vi "Configure SMU.vi"(5 "aperture time":dbl=0.001, 7 "Source Mode":enum16{"Voltage", "Current"}(ring), 8 "error in (no error)":errorcluster, 9 "Settings":T2 {"Sense" items=["Local"=1008, "Remote"=1009]}, 10 "Pins":string[](array[string]), 11 "Semiconductor Module Context":T3) -> (0 "error out":errorcluster)   [LabVIEW 2013]
uses:
  <vilib>/NI_TestStand_SemiconductorModule/NI_TestStand_Semiconductor_Module.lvlibp/PinMap/General/SemiconductorModuleContext.ctl
  <instrlib>/niDCPower/nidcpower.llb/niDCPower Sense.ctl
  <instrlib>/niDCPower/nidcpower.llb/niDCPower Aperture Time Units.ctl
  <instrlib>/niDCPower/nidcpower.llb/niDCPower Output Function.ctl
  <vilib>/NI_TestStand_SemiconductorModule/NI_TestStand_Semiconductor_Module.lvlibp/PinMap/DC Power/PinsToNIDCPowerSessions.vi
  <vilib>/NI_TestStand_SemiconductorModule/NI_TestStand_Semiconductor_Module.lvlibp
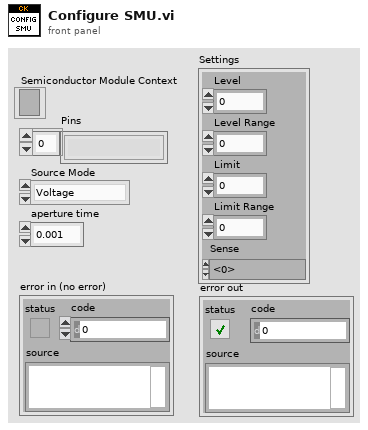
[diagram p1: front panel]
types:
  T1 = typedef "niDCPower Sense.ctl" = i32
  T2 = cluster{"Level":dbl, "Level Range":dbl, "Limit":dbl, "Limit Range":dbl, "Sense":T1}
  T3 = typedef "NI_TestStand_Semiconductor_Module.lvlibp/SemiconductorModuleContext.ctl" = refnum<k7>
  T4 = typedef "niDCPower Aperture Time Units.ctl" = i32
  T5 = typedef "niDCPower Output Function.ctl" = i32
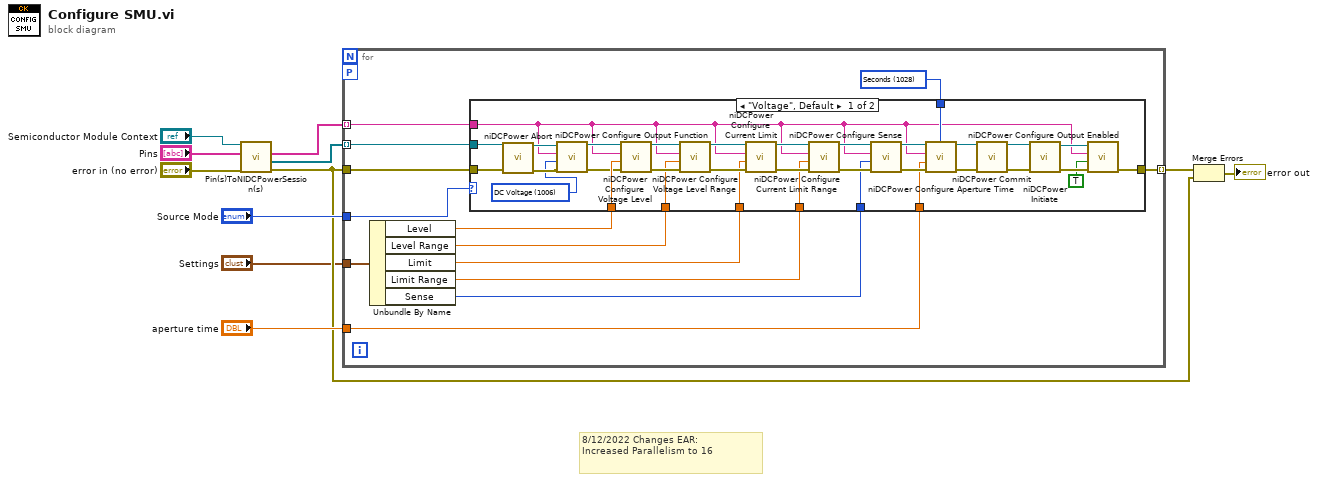
[diagram p0: block diagram]
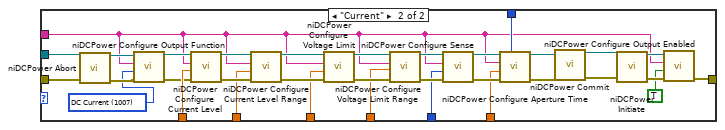
[diagram p2: hidden frame]
diagram:
  # "8/12/2022 Changes EAR:\nIncreased Parallelism to 16"
  n1 = call-poly <vilib>:"Pin(s)ToNIDCPowerSession(s).vi"("error in (no error)"="error in (no error)", "Pins"="Pins", "Semiconductor Module Context"="Semiconductor Module Context") -> ("error out"=w3:errorcluster, "Instrument Sessions"=w9:refnum<k15>[], "Channel Lists"=w8:string[])  [unwired: 4 in, 2 out]
  n2 = for {
    tunnel: w9 -> [w23] mode=indexing
    tunnel: w8 -> [w22] mode=indexing
    tunnel: "Settings" -> [w20]
    tunnel: "Source Mode" -> [w15]
    tunnel: "aperture time" -> [w12]
    tunnel: w3 -> [w24]
    tunnel: [w21] -> w5 mode=indexing
    workers-P: _ -> [_]
    w13 = T4 1028 items=["Seconds"=1028, "Powerline Cycles"=1029] ("aperture time units")
    n3 = Unbundle By Name(w20) -> ("Level"=w19:dbl, "Level Range"=w18:dbl, "Limit"=w17:dbl, "Limit Range"=w16:dbl, "Sense"=w14:T1)
    n4 = case shown="\"Voltage\", Default" w15 {
      tunnel: w24 -> [w31 w73]
      tunnel: w23 -> [w33 w72]
      tunnel: w22 -> [w26 w59]
      tunnel: [w28 w60] -> w21
      tunnel: w19 -> [w49 w90]
      tunnel: w18 -> [w48 w87]
      tunnel: w17 -> [w47 w84]
      tunnel: w16 -> [w46 w81]
      tunnel: w14 -> [w41 w78]
      tunnel: w12 -> [w43 w75]
      tunnel: w13 -> [w42 w74]
      frame "Voltage", Default {
        w34 = T5 1006 items=["DC Voltage"=1006, "DC Current"=1007, "Pulse Voltage"=1049, "Pulse Current"=1050] ("output function")
        n5 = call <instrlib>:"niDCPower Abort.vi"("error in (no error)"=w31, "instrument handle"=w33) -> ("error out"=w36:errorcluster, "instrument handle out"=w35:refnum<k15>)  [unwired: 8 in]
        n6 = call <instrlib>:"niDCPower Configure Output Function.vi"("error in (no error)"=w36, "output function"=w34, "channel name"=w26, "instrument handle"=w35) -> ("error out"=w30:errorcluster, "instrument handle out"=w32:refnum<k15>)  [unwired: 6 in]
        n7 = call <instrlib>:"niDCPower Configure Voltage Level.vi"("error in (no error)"=w30, "voltage level"=w49, "channel name"=w26, "instrument handle"=w32) -> ("error out"=w57:errorcluster, "instrument handle out"=w56:refnum<k15>)  [unwired: 6 in]
        n8 = call <instrlib>:"niDCPower Configure Voltage Level Range.vi"("error in (no error)"=w57, "voltage level range"=w48, "channel name"=w26, "instrument handle"=w56) -> ("error out"=w55:errorcluster, "instrument handle out"=w53:refnum<k15>)  [unwired: 6 in]
        n9 = call <instrlib>:"niDCPower Configure Current Limit.vi"("error in (no error)"=w55, "current limit"=w47, "channel name"=w26, "instrument handle"=w53) -> ("error out"=w54:errorcluster, "instrument handle out"=w52:refnum<k15>)  [unwired: 6 in]
        n10 = call <instrlib>:"niDCPower Configure Current Limit Range.vi"("error in (no error)"=w54, "current limit range"=w46, "channel name"=w26, "instrument handle"=w52) -> ("error out"=w51:errorcluster, "instrument handle out"=w50:refnum<k15>)  [unwired: 6 in]
        n11 = call <instrlib>:"niDCPower Configure Sense.vi"("error in (no error)"=w51, "sense"=w41, "channel name"=w26, "instrument handle"=w50) -> ("error out"=w45:errorcluster, "instrument handle out"=w44:refnum<k15>)  [unwired: 6 in]
        n12 = call <instrlib>:"niDCPower Configure Aperture Time.vi"("aperture time units"=w42, "error in (no error)"=w45, "aperture time"=w43, "channel name"=w26, "instrument handle"=w44) -> ("error out"=w39:errorcluster, "instrument handle out"=w40:refnum<k15>)  [unwired: 5 in]
        n13 = call <instrlib>:"niDCPower Commit.vi"("error in (no error)"=w39, "instrument handle"=w40) -> ("error out"=w38:errorcluster, "instrument handle out"=w37:refnum<k15>)  [unwired: 8 in]
        n14 = call <instrlib>:"niDCPower Initiate.vi"("error in (no error)"=w38, "instrument handle"=w37) -> ("error out"=w29:errorcluster, "instrument handle out"=w27:refnum<k15>)  [unwired: 8 in]
        n15 = call <instrlib>:"niDCPower Configure Output Enabled.vi"("error in (no error)"=w29, "output enabled"=TRUE, "channel name"=w26, "instrument handle"=w27) -> ("error out"=w28:errorcluster)  [unwired: 6 in, 1 out]
      }
      frame "Current" {
        w67 = T5 1007 items=["DC Voltage"=1006, "DC Current"=1007, "Pulse Voltage"=1049, "Pulse Current"=1050] ("output function")
        n16 = call <instrlib>:"niDCPower Abort.vi"("error in (no error)"=w73, "instrument handle"=w72) -> ("error out"=w69:errorcluster, "instrument handle out"=w68:refnum<k15>)  [unwired: 8 in]
        n17 = call <instrlib>:"niDCPower Configure Output Function.vi"("error in (no error)"=w69, "output function"=w67, "channel name"=w59, "instrument handle"=w68) -> ("error out"=w71:errorcluster, "instrument handle out"=w70:refnum<k15>)  [unwired: 6 in]
        n18 = call <instrlib>:"niDCPower Configure Current Level.vi"("error in (no error)"=w71, "current level"=w90, "channel name"=w59, "instrument handle"=w70) -> ("error out"=w89:errorcluster, "instrument handle out"=w88:refnum<k15>)  [unwired: 6 in]
        n19 = call <instrlib>:"niDCPower Configure Current Level Range.vi"("error in (no error)"=w89, "current level range"=w87, "channel name"=w59, "instrument handle"=w88) -> ("error out"=w86:errorcluster, "instrument handle out"=w85:refnum<k15>)  [unwired: 6 in]
        n20 = call <instrlib>:"niDCPower Configure Voltage Limit.vi"("error in (no error)"=w86, "voltage limit"=w84, "channel name"=w59, "instrument handle"=w85) -> ("error out"=w83:errorcluster, "instrument handle out"=w82:refnum<k15>)  [unwired: 6 in]
        n21 = call <instrlib>:"niDCPower Configure Voltage Limit Range.vi"("error in (no error)"=w83, "voltage limit range"=w81, "channel name"=w59, "instrument handle"=w82) -> ("error out"=w80:errorcluster, "instrument handle out"=w79:refnum<k15>)  [unwired: 6 in]
        n22 = call <instrlib>:"niDCPower Configure Sense.vi"("error in (no error)"=w80, "sense"=w78, "channel name"=w59, "instrument handle"=w79) -> ("error out"=w77:errorcluster, "instrument handle out"=w76:refnum<k15>)  [unwired: 6 in]
        n23 = call <instrlib>:"niDCPower Configure Aperture Time.vi"("aperture time units"=w74, "error in (no error)"=w77, "aperture time"=w75, "channel name"=w59, "instrument handle"=w76) -> ("error out"=w66:errorcluster, "instrument handle out"=w65:refnum<k15>)  [unwired: 5 in]
        n24 = call <instrlib>:"niDCPower Commit.vi"("error in (no error)"=w66, "instrument handle"=w65) -> ("error out"=w63:errorcluster, "instrument handle out"=w64:refnum<k15>)  [unwired: 8 in]
        n25 = call <instrlib>:"niDCPower Initiate.vi"("error in (no error)"=w63, "instrument handle"=w64) -> ("error out"=w62:errorcluster, "instrument handle out"=w61:refnum<k15>)  [unwired: 8 in]
        n26 = call <instrlib>:"niDCPower Configure Output Enabled.vi"("error in (no error)"=w62, "output enabled"=TRUE, "channel name"=w59, "instrument handle"=w61) -> ("error out"=w60:errorcluster)  [unwired: 6 in, 1 out]
      }
    }
  }
  n27 = Merge Errors(w5, w3) -> (→"error out":errorcluster)
